vi "_LVCMPlugin_IsSupportingItem.vi"(8 "error in (no error)":errorcluster, 9 "VI Reference":refnum<vi>, 10 "ProjectItem Refnum":refnum<vi>, 11 "_Default in":refnum<class "ClassMethodsInheritance.lvclass">) -> (0 "error out":errorcluster, 2 "IsSupportingItem":bool, 3 "_Default out":refnum<class "ClassMethodsInheritance.lvclass">)   [LabVIEW 2013, in "ClassMethodsInheritance.lvclass"]
uses:
  ClassMethodsInheritance.lvclass
  <resource>/Framework/Providers/Veritech_LVCM/Support/Utilites/_ProjectItemsUtilities/_ProjectItemsUtilities.lvlib
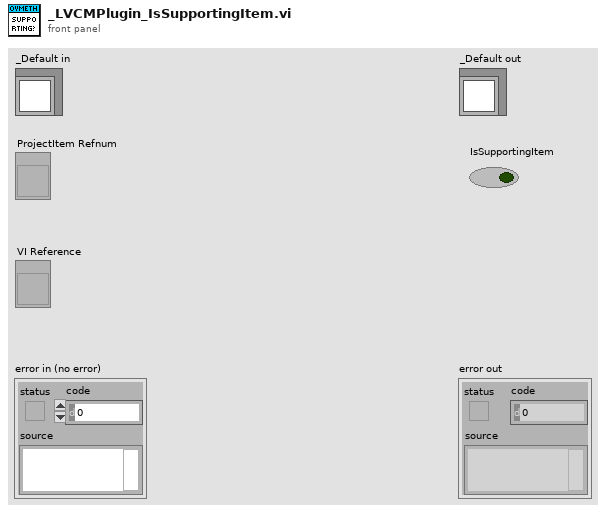
[diagram p1: front panel]
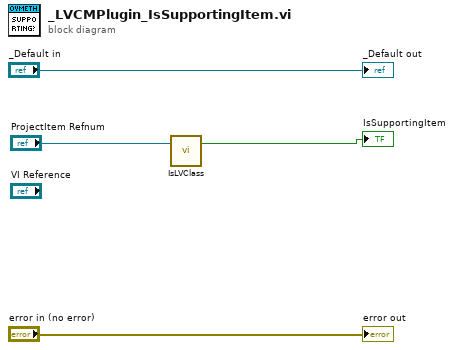
[diagram p0: block diagram]
diagram:
  n1 = call <resource>:"IsLVClass.vi"("ProjectItem Refnum"="ProjectItem Refnum") -> ("IsLVClass?"=→"IsSupportingItem":bool)  [unwired: 2 in]
  "error out" <- "error in (no error)"
  "_Default out" <- "_Default in"
